vi "TecanCarvroPump_Couple.vi"   [LabVIEW 2023]
types:
  T1 = enum16{"Initialize", "Absolute Position", "Relative Pickup", "Relative Dispense", "Swich valve", "Bypass"}
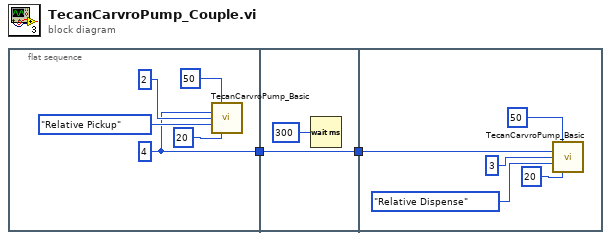
[diagram p0: block diagram]
diagram:
  n1 = flat-sequence {
    tunnel: [w3] -> w1
    tunnel: [w8] -> w2
    tunnel: w1 -> [w8]
    tunnel: w2 -> [w10]
    frame #0 {
      w3 = u8 4 ("TecanPump address")
      n2 = call "TecanCarvroPump_Basic.vi"("Volume (μL)"=u16 50, "TecanPump address"=w3, "Valve"=u8 2, "Mode"=T1."Relative Pickup", "Speed (μL/s)"=u16 20) -> ()  [unwired: 10 in, 1 out]
    }
    frame #1 {
      n3 = Wait (ms)(milliseconds to wait=u32 300) -> ()  [unwired: 1 out]
    }
    frame #2 {
      n4 = call "TecanCarvroPump_Basic.vi"("Volume (μL)"=u16 50, "TecanPump address"=w10, "Valve"=u8 3, "Mode"=T1."Relative Dispense", "Speed (μL/s)"=u16 20) -> ()  [unwired: 10 in, 1 out]
    }
  }
